vi "custom scale test.vi"(8 "error in":errorcluster) -> (0 "error out":errorcluster, 3 "task out":refnum<k21>)   [LabVIEW 2013]
uses:
  <vilib>/DAQmx/configure/timing.llb/DAQmx Timing (Sample Clock).vi
  <vilib>/DAQmx/create/channels.llb/DAQmx Create Channel (AI-Current-Basic).vi
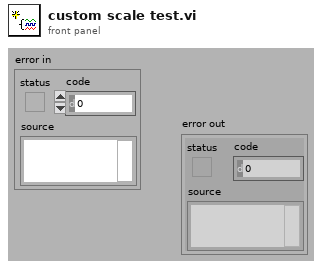
[diagram p1: front panel]
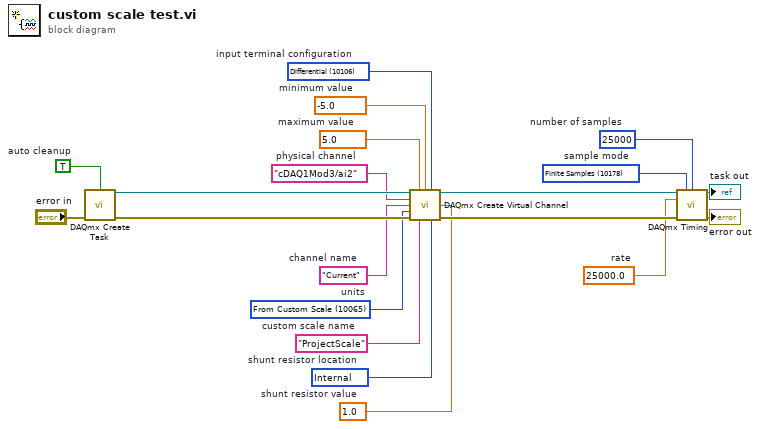
[diagram p0: block diagram]
diagram:
  w1 = 10178 items=["Finite Samples"=10178, "Continuous Samples"=10123, "Hardware Timed Single Point"=12522]  # sample mode
  w2 = 25000  # number of samples
  w3 = 25000.0  # rate
  w7 = 10106 items=["default"=-1, "RSE"=10083, "NRSE"=10078, "Differential"=10106, "Pseudodifferential"=12529]  # input terminal configuration
  w8 = 10065 items=["Amps"=10342, "From Custom Scale"=10065]  # units
  w9 = 1.0  # shunt resistor value
  w10 = 10200 items=["Internal"=10200, "External"=10167]  # shunt resistor location
  w11 = "Current"  # channel name
  w13 = "ProjectScale"  # custom scale name
  w14 = -5.0  # minimum value
  w15 = 5.0  # maximum value
  w16 = "cDAQ1Mod3/ai2"  # physical channel
  w18 = TRUE  # auto cleanup
  n1 = call <vilib>:"DAQmx Create Task.vi"("auto cleanup"=w18, "error in"="error in") -> ("task out"=w17:refnum<k21>, "error out"=w19:errorcluster)  [unwired: 12 in]
  n2 = call-poly <vilib>:"DAQmx Create Virtual Channel.vi"("task in"=w17, "maximum value"=w15, "minimum value"=w14, "input terminal configuration"=w7, "physical channels"=w16, "name to assign"=w11, "external shunt resistor value"=w9, "units"=w8, "error in"=w19, "custom scale name"=w13, "shunt resistor location"=w10) -> ("task out"=w4:refnum<k21>, "error out"=w12:errorcluster)  [unwired: 3 in]
  n3 = call-poly <vilib>:"DAQmx Timing.vi"("task/channels in"=w4, "sample mode"=w1, "samples per channel"=w2, "rate"=w3, "error in"=w12) -> ("task out"=→"task out":refnum<k21>, "error out"=→"error out":errorcluster)  [unwired: 9 in]
